vi "MAIN_HGB2_rev03.vi"() -> ()   [LabVIEW 2016]
uses:
  Producer_Case_Structure.ctl
  Consumer Control.ctl
  <vilib>/Utility/error.llb/DialogType.ctl
  <vilib>/DAQmx/write.llb/DAQmx Write (Analog 1D DBL NChan 1Samp).vi
  <vilib>/DAQmx/miscellaneous.llb/DAQmx Fill In Error Info.vi
  <vilib>/express/express analysis/Spectral/Block/exnSpectralBlock spectral measurements RMS poly.vi
  <vilib>/express/express analysis/Spectral/Block/exnSpectralBlock spectral measurements RMS array WFM.vi
  <vilib>/express/express analysis/Spectral/XNode/ExpressSpectralMeasurementsBlockNode.xnode
panel:
  in  "Dummy Variable 2":dbl=100.0
  in  "VFD On/Off":bool
  out "TDMS":i32=31
  out "Acc":i32
  in  "Numeric":i32
  out "Producer":i32=452
  out "Control":i32=10
  in  "Speed Setpoint":dbl
  in  "Operator Notes":string
  in  "Dummy Variable":dbl
  in  "Record Data":bool
  in  "Sample Rate [S/s]":dbl=10.0
  in  "file path":path=path "S:/002 - Projects/200804 AECSSB/6-Testing/TDMS Data/raw/JunkData/082621-ShutdownCheck4"
  in  "Stop":bool
  in  "Tab Control":T1(tab)=enum."Pressure & Temperature"
  out "System Temperatures":waveform(dbl)[](graph)=[{"t0"=timestamp(3712839887.203294 s since 1904-01-01), "dt"=0.1, "Y"=[25.650665015231628, 25.650665015231628, 25.650665015231628, 25.650094032394826, 25.650094032394826], "attributes"=variant("NI_ChannelName"=variant(string "T_dis_dwnstrm"), "NI_UnitDescription"=variant(string "Deg C"))}, {"t0"=timestamp(3712839887.203294 s since 1904-01-01), "dt"=0.1, "Y"=[21.37303402901582, 21.37303402901582, 21.37303402901582, 21.36692834475169, 21.36692834475169], "attributes"=variant("NI_ChannelName"=variant(string "T_liq"), "NI_UnitDescription"=variant(string "Deg C"))}, {"t0"=timestamp(3712839887.203294 s since 1904-01-01), "dt"=0.1, "Y"=[25.051178589493077, 25.051178589493077, 25.051178589493077, 25.046720547133443, 25.046720547133443], "attributes"=variant("NI_ChannelName"=variant(string "T_gas_mix"), "NI_UnitDescription"=variant(string "Deg C"))}, {"t0"=timestamp(3712839887.203294 s since 1904-01-01), "dt"=0.1, "Y"=[15.28260420449759, 15.28260420449759, 15.28260420449759, 15.302095088188059, 15.302095088188059], "attributes"=variant("NI_ChannelName"=variant(string "T_wf_cd_out"), "NI_UnitDescription"=variant(string "Deg C"))}, {"t0"=timestamp(3712839887.203294 s since 1904-01-01), "dt"=0.1, "Y"=[17.854844556084544, 17.854844556084544, 17.854844556084544, 17.936201243083087, 17.936201243083087], "attributes"=variant("NI_ChannelName"=variant(string "T_cf_in"), "NI_UnitDescription"=variant(string "Deg C"))}]
  out "System Pressures":waveform(dbl)[](graph)=[{"t0"=timestamp(3712839887.203294 s since 1904-01-01), "dt"=0.1, "Y"=[497.9062778476196, 497.9617200549117, 497.9593536192346, 497.9556349345991, 497.93366088902604], "attributes"=variant("NI_ChannelName"=variant(string "P_comp_suc"))}, {"t0"=timestamp(3712839887.203294 s since 1904-01-01), "dt"=0.1, "Y"=[500.46360622081005, 500.48118547426617, 500.5396702982644, 500.502145353387, 500.5122872303809], "attributes"=variant("NI_ChannelName"=variant(string "P_comp_dis"))}, {"t0"=timestamp(3712839887.203294 s since 1904-01-01), "dt"=0.1, "Y"=[498.7526715719359, 498.6975673736022, 498.7459103206066, 498.7313736302486, 498.67626943191505], "attributes"=variant("NI_ChannelName"=variant(string "P_comp_int"))}]
  out "Mass Flow":waveform(dbl)(graph)={"t0"=timestamp(3712839887.203294 s since 1904-01-01), "dt"=0.1, "Y"=[-2.5258889253594596e-05, -2.5376565371472426e-05, -2.545011294514607e-05, -2.5361855856737697e-05, -2.5361855856737697e-05], "attributes"=variant("NI_ChannelName"=variant(string "m_dot_wf"))}
  out "Setpoint Temperatures":waveform(dbl)[](graph)=[{"t0"=timestamp(3712839887.203294 s since 1904-01-01), "dt"=0.1, "Y"=[26.12327874474579, 26.12327874474579, 26.12327874474579, 26.12567352372733, 26.12567352372733], "attributes"=variant("NI_ChannelName"=variant(string "T_comp_suc"), "NI_UnitDescription"=variant(string "Deg C"))}, {"t0"=timestamp(3712839887.203294 s since 1904-01-01), "dt"=0.1, "Y"=[25.833285073903582, 25.833285073903582, 25.833285073903582, 25.830203756237246, 25.830203756237246], "attributes"=variant("NI_ChannelName"=variant(string "T_comp_out"), "NI_UnitDescription"=variant(string "Deg C"))}, {"t0"=timestamp(3712839887.203294 s since 1904-01-01), "dt"=0.1, "Y"=[10.549528033625506, 10.546050512616432, 10.546198937365375, 10.548826956323552, 10.550205219635103], "attributes"=variant("NI_ChannelName"=variant(string "Suc_Suph"), "NI_UnitDescription"=variant(string "Deg C"))}]
  out "Power Constituents":waveform(dbl)[](graph)=[{"t0"=timestamp(3712839887.203294 s since 1904-01-01), "dt"=0.1, "Y"=[-0.25374797068745636, -0.25404216098215215, -0.25404216098215215, -0.2541402244137174, -0.2541402244137174], "attributes"=variant("NI_ChannelName"=variant(string "Voltage"))}, {"t0"=timestamp(3712839887.203294 s since 1904-01-01), "dt"=0.1, "Y"=[-0.030598737819417465, -0.031007335450937035, -0.031203462314064012, -0.031154430598284932, -0.0311053988825023], "attributes"=variant("NI_ChannelName"=variant(string "Frequency"))}, {"t0"=timestamp(3712839886.9042945 s since 1904-01-01), "dt"=0.1, "Y"=[0.03397996537387371, 0.003032894805073738, -0.007282795384526253, -0.0021249502897262573, -0.012440640479326248], "attributes"=variant("NI_ChannelName"=variant(string "Torque"))}, {"t0"=timestamp(3712839886.9542933 s since 1904-01-01), "dt"=0.1, "Y"=[-13.228808343410492, 7.40257203578949, 1.2131579220294952, -9.102532267570496, 9.465710073709488], "attributes"=variant("NI_ChannelName"=variant(string "Tachometer"))}]
  out "Raw Acceleration":waveform(dbl)[](graph)
  out "Accel. Spectrum":cluster{"f0":dbl, "df":dbl, "magnitude":dbl[]}[](graph)
  in  "?":path=path "C:/Users/ASITest/Desktop/REFPROP"
  in  "Working Fluid":string="R134A.FLD"
  # "Stop VI"
  # "Air Squared Hot Gas Bypass Test Stand"
  # "Point to where REFPROP is..."
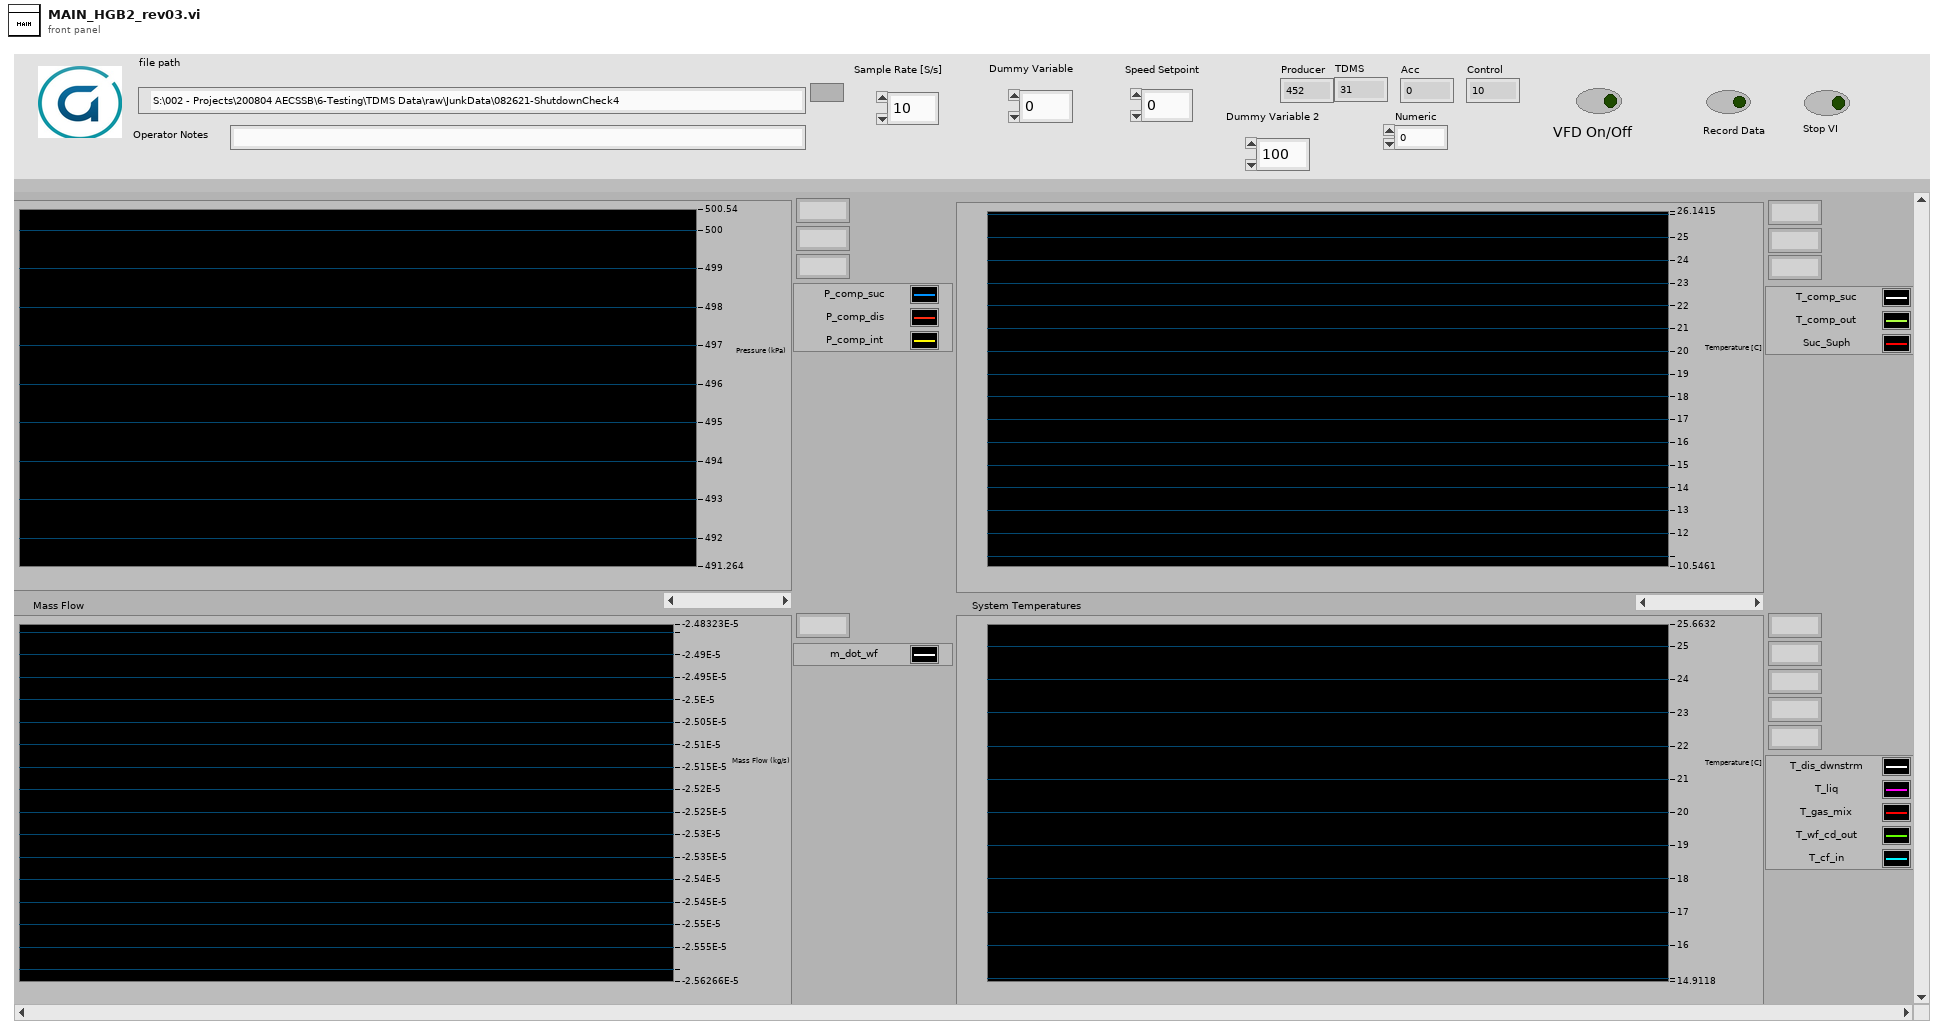
[diagram p1: front panel]
types:
  T1 = enum32{"Schematic", "Pressure & Temperature", "Power", "Acceleration", "Efficiency"}
  T2 = typedef "Consumer Control.ctl" = enum16{"System Run", "Shutdown"}
  T3 = enum16{"open", "open or create", "create or replace", "create", "open (read-only)"}
  T4 = typedef "Producer_Case_Structure.ctl" = enum16{"Initialize", "Read", "Write", "Display", "Queue", "Evaluate", "Error", "Shutdown"}
  T5 = cluster{"Data Main":waveform(dbl)[], "Accelerometer":waveform(dbl)[], "Dummy Variable":dbl, "Operator Notes":string, "Speed Setpoint":dbl, "NI 6001":waveform(dbl)[], "On/Off":dbl}
  T6 = typedef "DialogType.ctl" = u16
  T7 = cluster{"averaging mode":u16, "weighting mode":u16, "number of averages":u32}
  T8 = cluster{"dB On (F)":bool, "unwrap phase (F)":bool, "convert to degree (F)":bool}
  T9 = cluster{"All Channels":tag[], "All Labels":string[], "All Units":string[], "Slope":dbl[], "Y-Intercept":dbl[]}
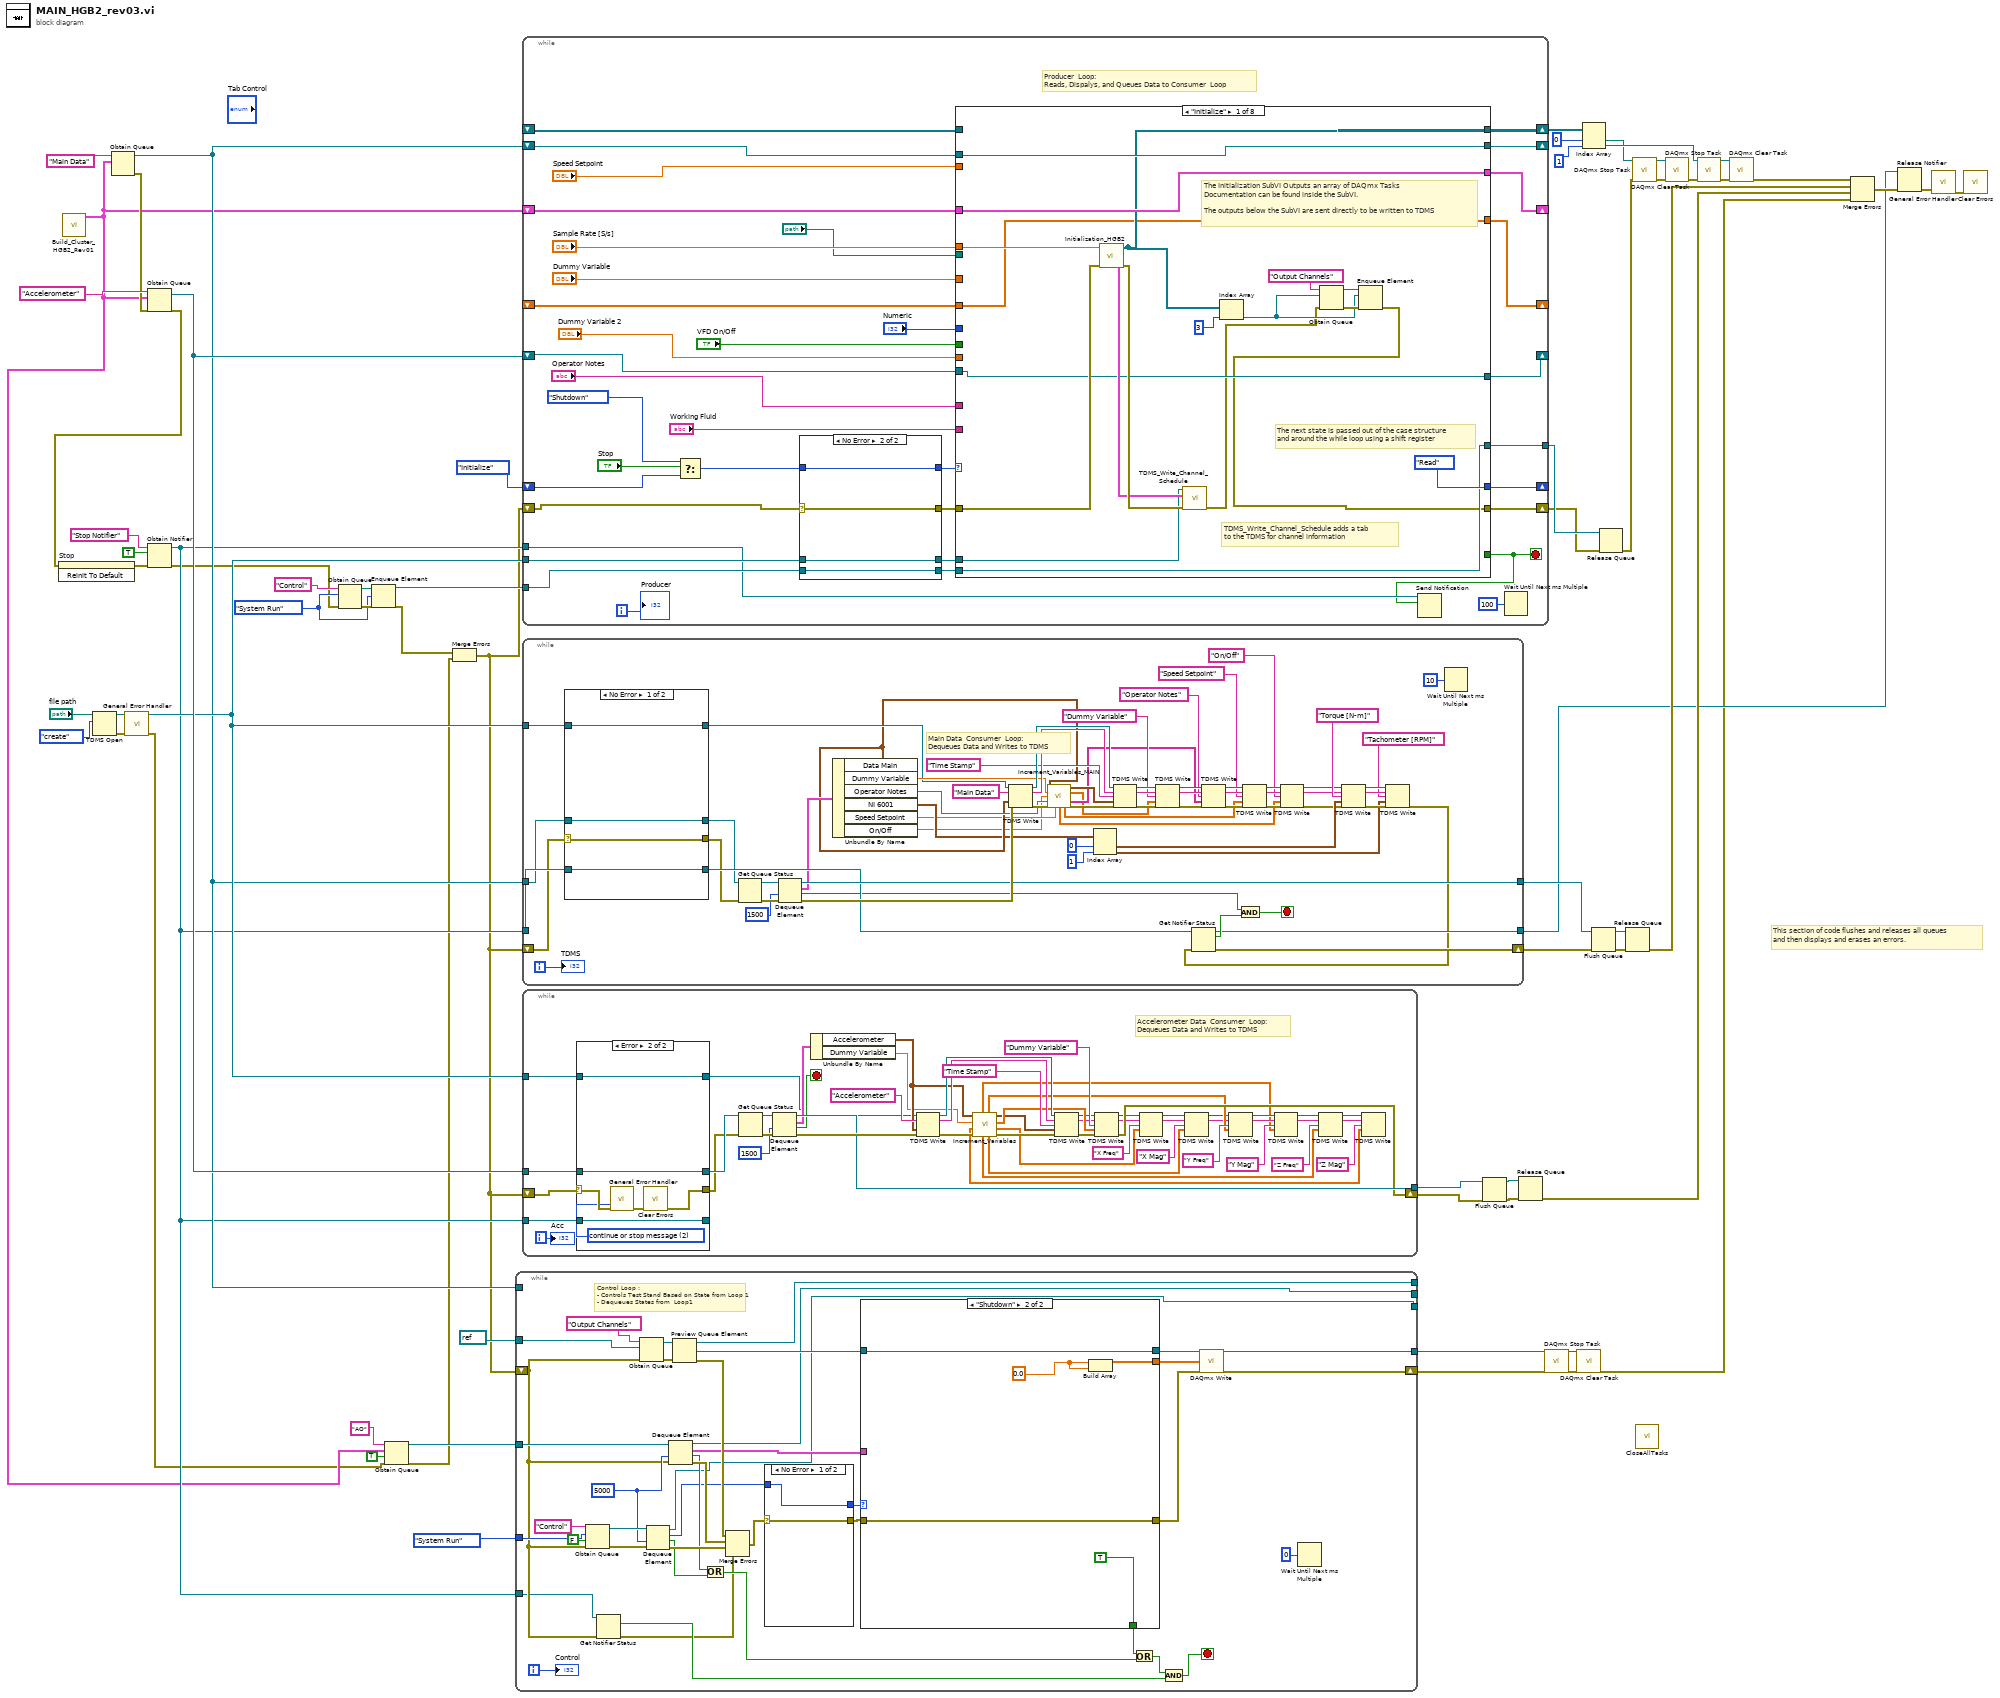
[diagram p0: block diagram]
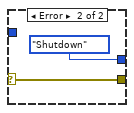
[diagram p2: hidden frame]
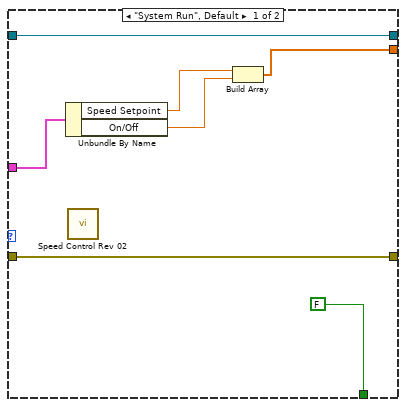
[diagram p3: hidden frame]
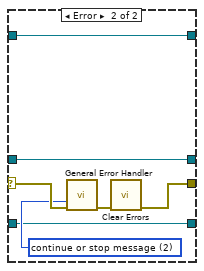
[diagram p5: hidden frame]
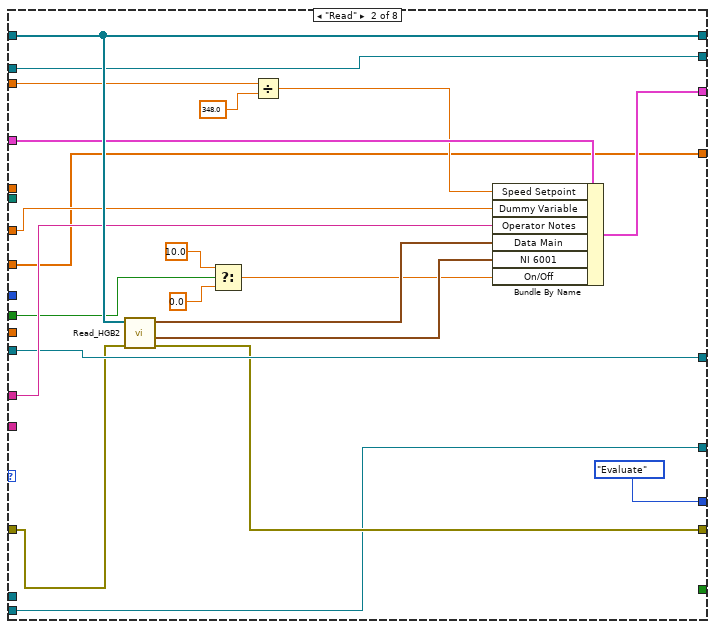
[diagram p6: hidden frame]
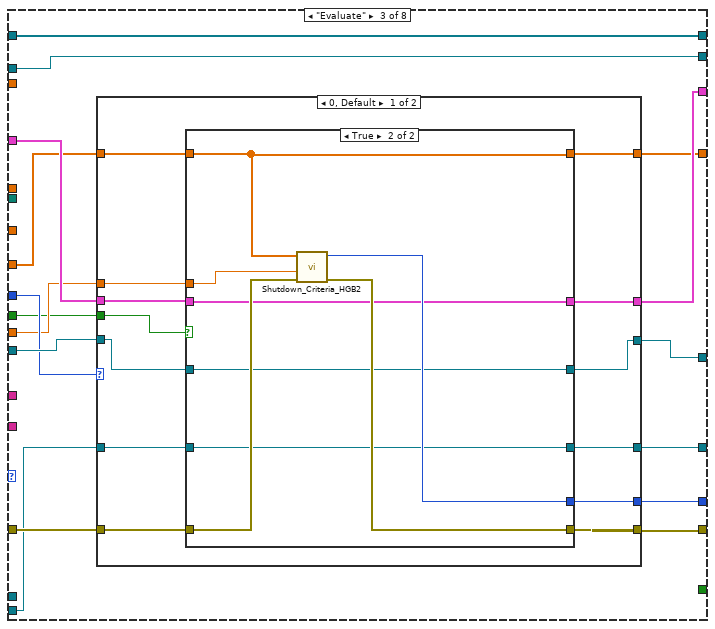
[diagram p7: hidden frame]
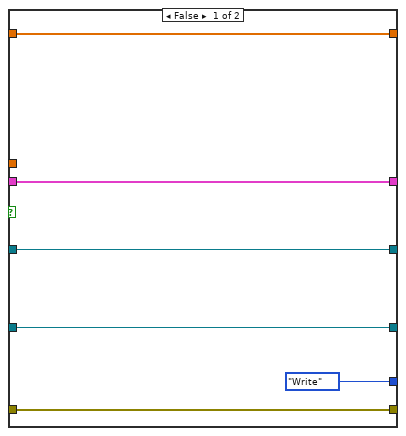
[diagram p8: hidden frame]
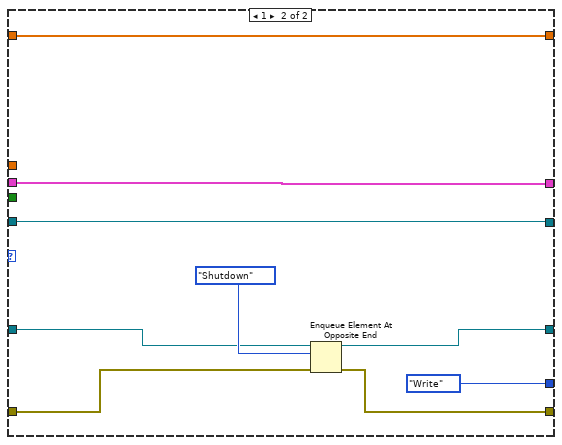
[diagram p9: hidden frame]
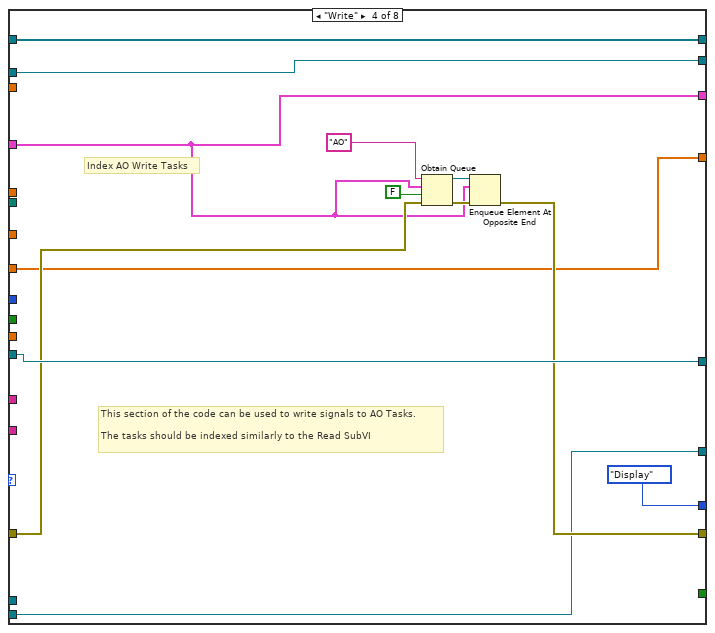
[diagram p10: hidden frame]
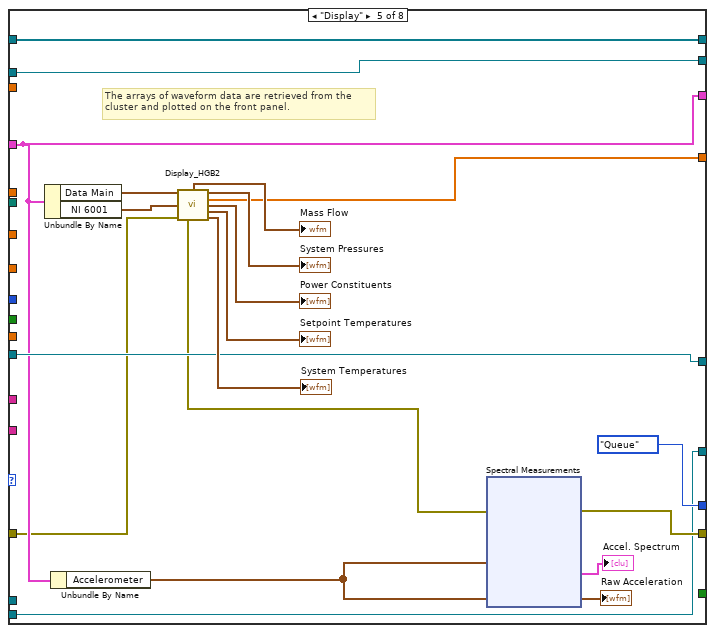
[diagram p11: hidden frame]
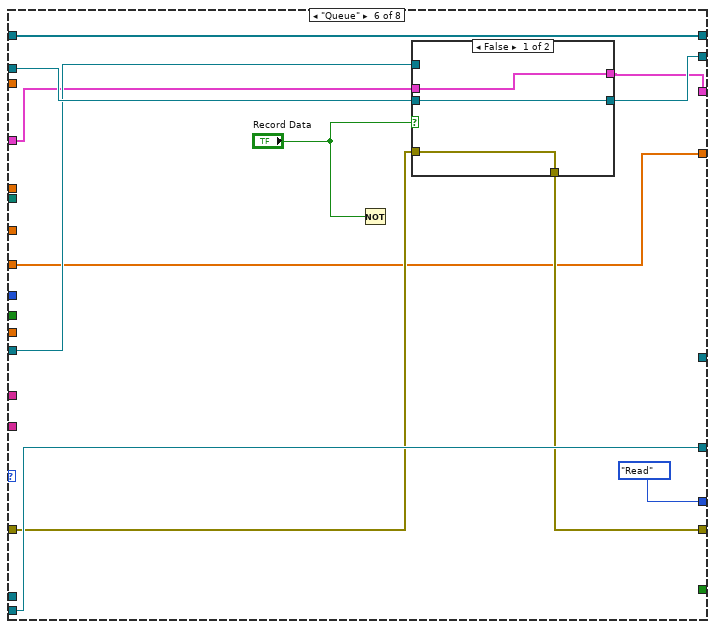
[diagram p12: hidden frame]
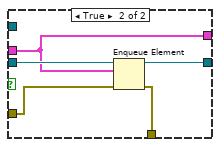
[diagram p13: hidden frame]
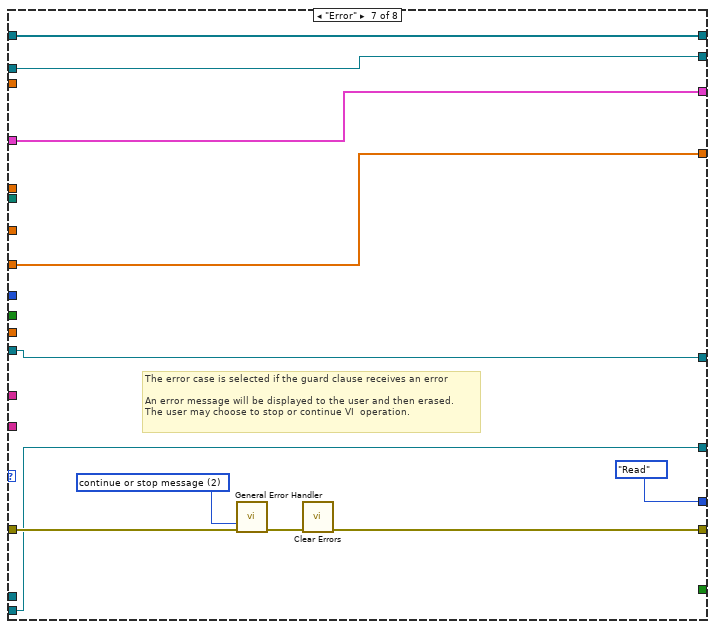
[diagram p14: hidden frame]
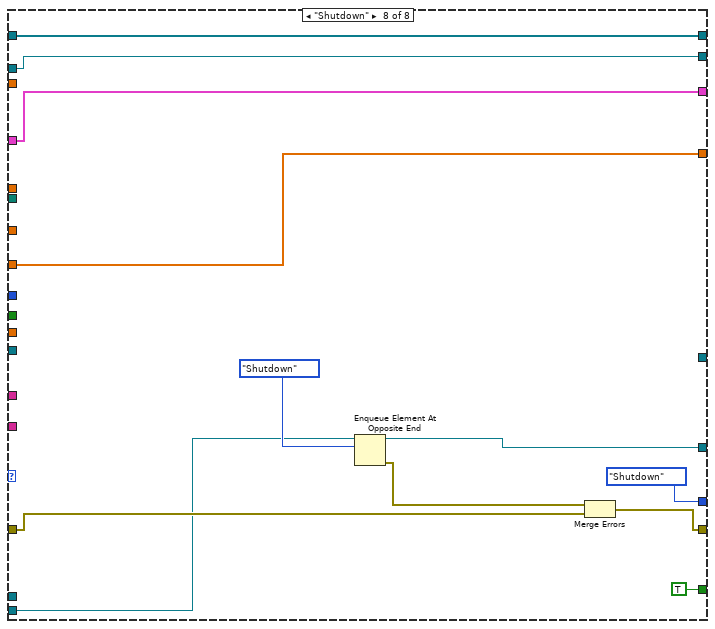
[diagram p15: hidden frame]
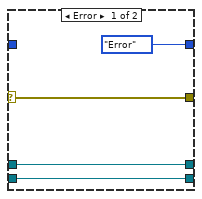
[diagram p16: hidden frame]
diagram:
  w21 = Consumer_Control."System Run"
  # "This section of code flushes and releases all queues \nand then displays and erases an errors."
  n1 = call "Build_Cluster_HGB2_Rev01.vi"() -> ("output cluster"=w13:T5)  [unwired: 11 in]
  n2 = TDMS Open(10:T3."create" ("operation (0:open)"), 11:"file path") -> (0:w54:errorcluster, 3:w37:refnum<k34>)  [unwired: 5 in]
  n3 = Obtain Queue(name (unnamed)="Main Data", element data type=w13) -> (queue out=w34:refnum<queue>, error out=w43:errorcluster)  [unwired: 3 in, 1 out]
  n4 = call <vilib>:"General Error Handler.vi"("error in (no error)"=w54) -> ("error out"=w12:errorcluster)  [unwired: 10 in, 4 out]
  n5 = Obtain Queue(name (unnamed)="Accelerometer", element data type=w13, error in (no error)=w43) -> (queue out=w42:refnum<queue>, error out=w11:errorcluster)  [unwired: 2 in, 1 out]
  n6 = invoke on="Stop" class="Bool (strict)" method="Reinit To Default"(error in=w11) -> (error out=w59:errorcluster)  [unwired: 2 in, 2 out]
  n7 = Obtain Notifier(name (unnamed)="Stop Notifier", notification data type=TRUE, error in (no error)=w59) -> (notifier out=w30:refnum<notifier>, error out=w10:errorcluster)  [unwired: 1 in, 1 out]
  n8 = Obtain Queue(name (unnamed)="Control", element data type=w21, error in (no error)=w10) -> (queue out=w23:refnum<queue>, error out=w22:errorcluster)  [unwired: 2 in, 1 out]
  n9 = Enqueue Element(queue=w23, element=w21, error in (no error)=w22) -> (queue out=w20:refnum<queue>, error out=w8:errorcluster)  [unwired: 1 in, 1 out]
  n10 = Obtain Queue(name (unnamed)="AO", element data type=w13, create if not found? (T)=TRUE, error in (no error)=w12) -> (queue out=w14:refnum<queue>, error out=w7:errorcluster)  [unwired: 1 in, 1 out]
  n11 = Merge Errors(w8, w7) -> (w9:errorcluster)
  n12 = while {
    tunnel: [w102] -> w4
    shift-right: [w89] -> w3
    shift-left: w9 -> [w70]
    tunnel: refnum<k21> refnum ("task in") -> [w97]
    tunnel: w34 -> [_]
    tunnel: Consumer_Control."System Run" -> [w87]
    tunnel: w30 -> [w69]
    tunnel: [w74] -> _
    tunnel: [w73] -> _
    tunnel: [w72] -> _
    tunnel: w14 -> [w71]
    i -> [w79]
    stop <- w68 stop-if-true
    w92 = 5000 ("timeout in ms (-1)")
    # "Control Loop :\n- Controls Test Stand Based on State from Loop 1\n- Dequeues States from  Loop1"
    n13 = Obtain Queue(name (unnamed)="Control", element data type=w87, create if not found? (T)=FALSE, error in (no error)=w70) -> (queue out=w101:refnum<queue>, error out=w93:errorcluster)  [unwired: 1 in, 1 out]
    n14 = Get Notifier Status(notifier=w69, error in (no error)=w70) -> (current notification=w66:bool, error out=w65:errorcluster)  [unwired: 3 out]
    n15 = Obtain Queue(name (unnamed)="Output Channels", element data type=w97, error in (no error)=w70) -> (queue out=w98:refnum<queue>, error out=w96:errorcluster)  [unwired: 2 in, 1 out]
    n16 = Dequeue Element(queue=w101, timeout in ms (-1)=w92, error in (no error)=w93) -> (queue out=w72:refnum<queue>, element=w86:T2, timed out?=w90:bool, error out=w94:errorcluster)
    n17 = Dequeue Element(queue=w71, timeout in ms (-1)=w92, error in (no error)=w70) -> (queue out=w73:refnum<queue>, element=w80:T5, timed out?=w91:bool, error out=w95:errorcluster)
    n18 = Preview Queue Element(queue=w98, error in (no error)=w96) -> (queue out=w74:refnum<queue>, element=w99:refnum<k21>, error out=w88:errorcluster)  [unwired: 1 in, 1 out]
    n19 = Or(x=w91, y=w90) -> (x .or. y?=w77:bool)
    n20 = Merge Errors(w88, w95, w94, w65) -> (w85:errorcluster)
    n21 = case shown="No Error" w85 {
      selector: w85 -> [w106 w108]
      tunnel: [w106 w108] -> w84
      tunnel: w86 -> [w105 _]
      tunnel: [w105 Consumer_Control."Shutdown"] -> w83
      frame No Error {
      }
      frame Error {
      }
    }
    n22 = case shown="\"Shutdown\"" w83 {
      tunnel: w99 -> [w115 w119]
      tunnel: [w110 w120] -> w104
      tunnel: [w115 w119] -> w103
      tunnel: w80 -> [w112 _]
      tunnel: w84 -> [w113 w117]
      tunnel: [FALSE TRUE] -> w78
      tunnel: [w113 w117] -> w82
      frame "System Run", Default {
        n23 = Unbundle By Name(w112) -> ("Speed Setpoint"=w111:dbl, "On/Off"=w109:dbl)
        n24 = call "Speed Control Rev 02.vi"() -> ()  [unwired: 11 in, 1 out]
        n25 = Build Array(w111, w109) -> (w110:dbl[])
      }
      frame "Shutdown" {
        w116 = 0.0 ("Speed Setpoint 2")
        n26 = Build Array(w116, w116) -> (w120:dbl[])
      }
    }
    n27 = Or(x=w78, y=w77) -> (x .or. y?=w67:bool)
    n28 = And(x=w67, y=w66) -> (x .and. y?=w68:bool)
    n29 = call-poly <vilib>:"DAQmx Write.vi"("task/channels in"=w103, "data"=w104, "error in"=w82) -> ("task out"=w102:refnum<k21>, "error out"=w89:errorcluster)  [unwired: 10 in, 1 out]
    n30 = Wait Until Next ms Multiple(millisecond multiple=u32 0) -> ()  [unwired: 1 out]
    "Control" <- w79
  }
  n31 = while {
    tunnel: w37 -> [w175]
    tunnel: [w185] -> w51
    tunnel: w34 -> [w176]
    tunnel: w30 -> [w178]
    shift-right: [w183] -> w26
    shift-left: w9 -> [w174]
    tunnel: [w153] -> w25
    i -> [w138]
    stop <- w180 stop-if-true
    # "Main Data  Consumer  Loop: \nDequeues Data and Writes to TDMS"
    n32 = case shown="No Error" w174 {
      selector: w174 -> [w191 w197]
      tunnel: [w191 w196] -> w156
      tunnel: w178 -> [w190 w192]
      tunnel: [w190 w192] -> w179
      tunnel: [w189 w194] -> w177
      tunnel: w176 -> [w189 w194]
      tunnel: [w188 w193] -> w154
      tunnel: w175 -> [w188 w193]
      frame No Error {
      }
      frame Error {
        w195 = T6 2 items=["no dialog", "OK message", "continue or stop message", "OK message + warnings", "continue/stop + warnings"] ("type of dialog (OK msg:1)")
        n33 = call <vilib>:"General Error Handler.vi"("type of dialog (OK msg:1)"=w195, "error in (no error)"=w197) -> ("error out"=w198:errorcluster)  [unwired: 9 in, 4 out]
        n34 = call <vilib>:"Clear Errors.vi"("error in (no error)"=w198) -> ("error out"=w196:errorcluster)  [unwired: 5 in, 1 out]
      }
    }
    n35 = Get Queue Status(queue=w177, error in (no error)=w156) -> (queue out=w182:refnum<queue>, error out=w186:errorcluster)  [unwired: 1 in, 6 out]
    n36 = Dequeue Element(queue=w182, timeout in ms (-1)=1500, error in (no error)=w186) -> (queue out=w185:refnum<queue>, element=w155:T5, timed out?=w173:bool, error out=w187:errorcluster)
    n37 = Unbundle By Name(w155) -> ("Data Main"=w145:waveform(dbl)[], "Dummy Variable"=w163:dbl, "Operator Notes"=w151:string, "NI 6001"=w140:waveform(dbl)[], "Speed Setpoint"=w139:dbl, "On/Off"=w123:dbl)
    n38 = TDMS Write(0:w154, 5:"Main Data" ("group name in (Untitled)"), 9:w145, 11:w187) -> (4:w170:refnum<k34>, 6:w168:string, 15:w171:errorcluster)  [unwired: 2 in, 1 out]
    n39 = call "Increment_Variables_MAIN.vi"("Data Main"=w145, "Dummy Variable"=w163, "On/Off"=w123, "Operator Notes"=w151, "error in 2"=w171, "Speed Setpoint"=w139) -> ("Time Stamp"=w164:timestamp[], "Dummy Variable Array"=w141:dbl[], "Operator Notes Array"=w152:string[], "On/Off Array"=w122:dbl[], "Speed Setpoint Array"=w147:dbl[], "error IO"=w172:errorcluster)  [unwired: 4 in]
    n40 = Index Array(array=w140, index #1=0 ("index"), index #2=1 ("index")) -> (element #1=w142:waveform(dbl), element #2=w130:waveform(dbl))
    n41 = TDMS Write(0:w170, 5:w168, 7:"Time Stamp" ("group name in (Untitled)"), 9:w164, 11:w172) -> (4:w167:refnum<k34>, 6:w165:string, 15:w166:errorcluster)  [unwired: 1 in, 1 out]
    n42 = TDMS Write(0:w167, 5:w165, 7:"Dummy Variable" ("group name in (Untitled)"), 9:w141, 11:w166) -> (4:w161:refnum<k34>, 6:w160:string, 15:w162:errorcluster)  [unwired: 1 in, 1 out]
    n43 = TDMS Write(0:w161, 5:w160, 7:"Operator Notes" ("group name in (Untitled)"), 9:w152, 11:w162) -> (4:w148:refnum<k34>, 6:w149:string, 15:w150:errorcluster)  [unwired: 1 in, 1 out]
    n44 = TDMS Write(0:w148, 5:w149, 7:"Speed Setpoint" ("group name in (Untitled)"), 9:w147, 11:w150) -> (4:w129:refnum<k34>, 6:w128:string, 15:w127:errorcluster)  [unwired: 1 in, 1 out]
    n45 = TDMS Write(0:w129, 5:w128, 7:"On/Off" ("channel name(s) in (Untitled)"), 9:w122, 11:w127) -> (4:w125:refnum<k34>, 6:w124:string, 15:w126:errorcluster)  [unwired: 1 in, 1 out]
    n46 = TDMS Write(0:w125, 5:w124, 7:"Torque [N-m]" ("channel name(s) in (Untitled)"), 9:w142, 11:w126) -> (4:w132:refnum<k34>, 6:w133:string, 15:w135:errorcluster)  [unwired: 1 in, 1 out]
    n47 = TDMS Write(0:w132, 5:w133, 7:"Tachometer [RPM]" ("channel name(s) in (Untitled)"), 9:w130, 11:w135) -> (15:w134:errorcluster)  [unwired: 1 in, 3 out]
    n48 = Get Notifier Status(notifier=w179, error in (no error)=w134) -> (notifier out=w153:refnum<notifier>, current notification=w184:bool, error out=w183:errorcluster)  [unwired: 2 out]
    n49 = And(x=w173, y=w184) -> (x .and. y?=w180:bool)
    n50 = Wait Until Next ms Multiple(millisecond multiple=u32 10) -> ()  [unwired: 1 out]
    "TDMS" <- w138
  }
  n51 = while {
    shift-right: [w230] -> _
    shift-left: Producer_Case_Structure."Initialize" ("Enum") -> [w209]
    shift-right: [w232] -> w56
    shift-left: _ -> [w231]
    tunnel: w30 -> [w206]
    shift-right: [w229] -> _
    shift-left: w13 -> [w228]
    shift-right: [w227] -> _
    shift-left: w34 -> [w226]
    shift-right: [w233] -> w18
    shift-left: w9 -> [w205]
    tunnel: w37 -> [w221]
    shift-right: [w219] -> _
    shift-left: w42 -> [w220]
    tunnel: w20 -> [w214]
    tunnel: [w212] -> w19
    shift-right: [w202] -> _
    shift-left: _ -> [w201]
    i -> [w215]
    stop <- w199 stop-if-true
    # "Producer  Loop: \nReads, Dispalys, and Queues Data to Consumer  Loop"
    n52 = Select(t=Producer_Case_Structure."Shutdown" ("Enum"), s="Stop", f=w209) -> (s? t:f=w208:T4)
    n53 = case shown="No Error" w205 {
      selector: w205 -> [w415 w420]
      tunnel: [w415 w420] -> w234
      tunnel: w208 -> [_ w419]
      tunnel: [Producer_Case_Structure."Error" ("Enum") w419] -> w235
      tunnel: [w414 w418] -> w222
      tunnel: w221 -> [w414 w418]
      tunnel: w214 -> [w413 w417]
      tunnel: [w413 w417] -> w213
      frame Error {
      }
      frame No Error {
      }
    }
    n54 = case shown="\"Initialize\"" w235 {
      tunnel: w234 -> [w254 w263 w289 w334 w344 w372 w397 w410]
      tunnel: [w237 w266 w288 w336 w352 w371 w394 w409] -> w233
      tunnel: [w242 w274 w284 w340 w358 w380 w398 w406] -> w232
      tunnel: w231 -> [_ w274 w284 w340 w358 w380 w398 w406]
      tunnel: [Producer_Case_Structure."Read" ("Enum") Producer_Case_Structure."Evaluate" ("Enum") w280 Producer_Case_Structure."Display" ("Enum") Producer_Case_Structure."Queue" ("Enum") Producer_Case_Structure."Read" ("Enum") Producer_Case_Structure."Read" ("Enum") Producer_Case_Structure."Shutdown" ("Enum")] -> w230
      tunnel: [_ _ _ _ _ _ _ TRUE ("Stop")] -> w199
      tunnel: [w250 w272 w290 w329 w351 w377 w396 w404] -> w229
      tunnel: w228 -> [w250 w268 w291 w329 w351 w375 w396 w404]
      tunnel: [w252 w273 w285 w338 w356 w378 w393 w405] -> w227
      tunnel: w226 -> [w252 w273 w285 w338 w356 w379 w393 w405]
      tunnel: "Sample Rate [S/s]" -> [w251 _ _ _ _ _ _ _]
      tunnel: "Dummy Variable" -> [_ w269 _ _ _ _ _ _]
      tunnel: "Operator Notes" -> [_ w271 _ _ _ _ _ _]
      tunnel: w222 -> [w247 _ _ _ _ _ _ _]
      tunnel: w220 -> [w246 w270 w283 w337 w354 w376 w392 _]
      tunnel: [w246 w270 w282 w337 w354 _ w392 _] -> w219
      tunnel: "?" -> [_ _ _ _ _ _ _ _]
      tunnel: "Working Fluid" -> [_ _ _ _ _ _ _ _]
      tunnel: "Speed Setpoint" -> [_ w257 _ _ _ _ _ _]
      tunnel: w213 -> [w239 w264 w287 w335 w343 w373 w391 w408]
      tunnel: [w239 w264 w286 w335 w343 w373 w391 w407] -> w212
      tunnel: "Numeric" -> [_ _ w281 _ _ _ _ _]
      tunnel: "VFD On/Off" -> [_ w260 w276 _ _ _ _ _]
      tunnel: [w236 w255 w278 w328 w342 w370 w390 w401] -> w202
      tunnel: w201 -> [w236 w255 w279 w328 _ w370 w390 w401]
      tunnel: "Dummy Variable 2" -> [_ _ w277 _ _ _ _ _]
      frame "Initialize" {
        # "TDMS_Write_Channel_Schedule adds a tab \nto the TDMS for channel information"
        # "The next state is passed out of the case structure \nand around the while loop using a shift register"
        # "The Initialization SubVI Outputs an array of DAQmx Tasks\nDocumentation can be found inside the SubVI.\n\nThe outputs below the SubVI are sent directly to be written to TDMS"
        n55 = call "Initialization_HGB2.vi"("error in"=w254, "Sample Rate"=w251) -> ("error out"=w249:errorcluster, "Task Array"=w242:refnum<k21>[], "output cluster"=w248:T9)  [unwired: 7 in]
        n56 = call "TDMS_Write_Channel_Schedule.vi"("error in (no error)"=w249, "output cluster"=w248, "Refnum in"=w247) -> ("error out"=w238:errorcluster)  [unwired: 8 in]
        n57 = Index Array(array=w242, index=3) -> (element=w240:refnum<k21>)
        n58 = Obtain Queue(name (unnamed)="Output Channels", element data type=w240, error in (no error)=w238) -> (queue out=w244:refnum<queue>, error out=w243:errorcluster)  [unwired: 2 in, 1 out]
        n59 = Enqueue Element(queue=w244, element=w240, error in (no error)=w243) -> (error out=w237:errorcluster)  [unwired: 1 in, 2 out]
      }
      frame "Read" {
        n60 = call "Read_HGB2.vi"("error in (no error)"=w263, "Task Array"=w274) -> ("error out"=w266:errorcluster, "NI 6001"=w265:waveform(dbl)[], "Data Main"=w267:waveform(dbl)[])  [unwired: 7 in]
        n61 = Select(t=10.0, s=w260, f=0.0) -> (s? t:f=w259:dbl)
        n62 = Divide(x=w257, y=348.0) -> (x/y=w256:dbl)
        n63 = Bundle By Name(cluster=w268, "Speed Setpoint"=w256, "Dummy Variable"=w269, "Operator Notes"=w271, "Data Main"=w267, "NI 6001"=w265, "On/Off"=w259) -> (w272:T5)
      }
      frame "Evaluate" {
        n64 = case shown="0, Default" w281 {
          tunnel: w291 -> [w300 w327]
          tunnel: [w299 w327] -> w290
          tunnel: w289 -> [w304 w323]
          tunnel: [w302 w322] -> w288
          tunnel: w287 -> [w293 w325]
          tunnel: [w292 w324] -> w286
          tunnel: [w298 w321] -> w282
          tunnel: w283 -> [w297 w321]
          tunnel: [w301 Producer_Case_Structure."Write" ("Enum")] -> w280
          tunnel: w279 -> [w294 w319]
          tunnel: [w295 w319] -> w278
          tunnel: w277 -> [w303 _]
          tunnel: w276 -> [w296 _]
          frame 0, Default {
            n65 = case shown="True" w296 {
              tunnel: w294 -> [w310 w312]
              tunnel: w304 -> [w307 w318]
              tunnel: w303 -> [_ w317]
              tunnel: [w307 w316] -> w302
              tunnel: [Producer_Case_Structure."Write" ("Enum") w315] -> w301
              tunnel: w300 -> [w309 w314]
              tunnel: [w309 w314] -> w299
              tunnel: [w308 w313] -> w298
              tunnel: w297 -> [w308 w313]
              tunnel: [w310 w312] -> w295
              tunnel: w293 -> [w306 w311]
              tunnel: [w306 w311] -> w292
              frame False {
              }
              frame True {
                n66 = call "Shutdown_Criteria_HGB2.vi"("error in (no error)"=w318, "Dummy Variable 2"=w317, "Data Array"=w312) -> ("error out"=w316:errorcluster, "Enum"=w315:T4)  [unwired: 7 in]
              }
            }
          }
          frame 1 {
            n67 = Enqueue Element At Opposite End(queue=w325, element=Consumer_Control."Shutdown", error in (no error)=w323) -> (queue out=w324:refnum<queue>, error out=w322:errorcluster)  [unwired: 1 in, 1 out]
          }
        }
      }
      frame "Write" {
        # "This section of the code can be used to write signals to AO Tasks.\n\nThe tasks should be indexed similarly to the Read SubVI"
        # "Index AO Write Tasks"
        n68 = Obtain Queue(name (unnamed)="AO", element data type=w329, create if not found? (T)=FALSE, error in (no error)=w334) -> (queue out=w332:refnum<queue>, error out=w333:errorcluster)  [unwired: 1 in, 1 out]
        n69 = Enqueue Element At Opposite End(queue=w332, element=w329, error in (no error)=w333) -> (error out=w336:errorcluster)  [unwired: 1 in, 2 out]
      }
      frame "Display" {
        # "The arrays of waveform data are retrieved from the \ncluster and plotted on the front panel."
        n70 = Unbundle By Name(w351) -> ("Data Main"=w349:waveform(dbl)[], "NI 6001"=w345:waveform(dbl)[])
        n71 = Unbundle By Name(w351) -> ("Accelerometer"=w350:waveform(dbl)[])
        "Raw Acceleration" <- w350
        n72 = call "Display_HGB2.vi"("data"=w349, "NI 6001"=w345, "error in (no error)"=w344) -> ("Mass Flow"=→"Mass Flow":waveform(dbl), "System Pressures"=→"System Pressures":waveform(dbl)[], "Data Array"=w342:dbl[], "Power Constituents"=→"Power Constituents":waveform(dbl)[], "Setpoint Temperatures"=→"Setpoint Temperatures":waveform(dbl)[], "error out"=w353:errorcluster, "System Temperatures"=→"System Temperatures":waveform(dbl)[])  [unwired: 6 in]
        n73 = xnode "Spectral Measurements"("Signals"=w350, "error in (no error)"=w353) -> ("FFT - (RMS)"=→"Accel. Spectrum":cluster{"f0":dbl, "df":dbl, "magnitude":dbl[]}[], "error out"=w352:errorcluster)  [unwired: 1 out]
      }
      frame "Queue" {
        n74 = Not(x="Record Data") -> ()  [unwired: 1 out]
        n75 = case shown="False" "Record Data" {
          tunnel: w375 -> [w383 w387]
          tunnel: w379 -> [w384 w388]
          tunnel: [w384 w389] -> w378
          tunnel: [w383 w387] -> w377
          tunnel: w376 -> [_ _]
          tunnel: w372 -> [w382 w386]
          tunnel: [w382 w385] -> w371
          frame False {
          }
          frame True {
            n76 = Enqueue Element(queue=w388, element=w387, error in (no error)=w386) -> (queue out=w389:refnum<queue>, error out=w385:errorcluster)  [unwired: 1 in, 1 out]
          }
        }
      }
      frame "Error" {
        w399 = T6 2 items=["no dialog", "OK message", "continue or stop message", "OK message + warnings", "continue/stop + warnings"] ("type of dialog (OK msg:1)")
        # "The error case is selected if the guard clause receives an error\n\nAn error message will be displayed to the user and then erased. \nThe user may choose to stop or continue VI  operation."
        n77 = call <vilib>:"General Error Handler.vi"("type of dialog (OK msg:1)"=w399, "error in (no error)"=w397) -> ("error out"=w395:errorcluster)  [unwired: 9 in, 4 out]
        n78 = call <vilib>:"Clear Errors.vi"("error in (no error)"=w395) -> ("error out"=w394:errorcluster)  [unwired: 5 in, 1 out]
      }
      frame "Shutdown" {
        n79 = Enqueue Element At Opposite End(queue=w408, element=Consumer_Control."Shutdown") -> (queue out=w407:refnum<queue>, error out=w411:errorcluster)  [unwired: 2 in, 1 out]
        n80 = Merge Errors(w411, w410) -> (w409:errorcluster)
      }
    }
    n81 = Send Notification(notification=w199, notifier=w206) -> ()  [unwired: 1 in, 2 out]
    n82 = Wait Until Next ms Multiple(millisecond multiple=u32 100) -> ()  [unwired: 1 out]
    "Producer" <- w215
  }
  n83 = while {
    tunnel: w37 -> [w466]
    tunnel: [w472] -> w39
    tunnel: w42 -> [w467]
    tunnel: w30 -> [w469]
    shift-right: [w447] -> w36
    shift-left: w9 -> [w465]
    i -> [w421]
    stop <- w446 stop-if-true
    # "Accelerometer Data  Consumer  Loop: \nDequeues Data and Writes to TDMS"
    n84 = case shown="Error" w465 {
      selector: w465 -> [w478 w484]
      tunnel: [w478 w483] -> w457
      tunnel: w469 -> [w477 w479]
      tunnel: [w477 w479] -> _
      tunnel: [w476 w481] -> w468
      tunnel: w467 -> [w476 w481]
      tunnel: [w475 w480] -> w455
      tunnel: w466 -> [w475 w480]
      frame No Error {
      }
      frame Error {
        w482 = T6 2 items=["no dialog", "OK message", "continue or stop message", "OK message + warnings", "continue/stop + warnings"] ("type of dialog (OK msg:1)")
        n85 = call <vilib>:"General Error Handler.vi"("type of dialog (OK msg:1)"=w482, "error in (no error)"=w484) -> ("error out"=w485:errorcluster)  [unwired: 9 in, 4 out]
        n86 = call <vilib>:"Clear Errors.vi"("error in (no error)"=w485) -> ("error out"=w483:errorcluster)  [unwired: 5 in, 1 out]
      }
    }
    n87 = Get Queue Status(queue=w468, error in (no error)=w457) -> (queue out=w471:refnum<queue>, error out=w473:errorcluster)  [unwired: 1 in, 6 out]
    n88 = Dequeue Element(queue=w471, timeout in ms (-1)=1500, error in (no error)=w473) -> (queue out=w472:refnum<queue>, element=w456:T5, timed out?=w446:bool, error out=w474:errorcluster)
    n89 = Unbundle By Name(w456) -> ("Accelerometer"=w459:waveform(dbl)[], "Dummy Variable"=w454:dbl)
    n90 = TDMS Write(0:w455, 5:"Accelerometer" ("group name in (Untitled)"), 9:w459, 11:w474) -> (4:w462:refnum<k34>, 6:w460:string, 15:w463:errorcluster)  [unwired: 2 in, 1 out]
    n91 = call "Increment_Variables.vi"("error in 2"=w463, "Dummy Variable"=w454, "Accelerometer"=w459) -> ("error IO"=w464:errorcluster, "X Accel Freq Array"=w443:dbl[], "Dummy Variable Array"=w452:dbl[], "Time Stamp"=w448:timestamp[], "X Accel Mag Array"=w441:dbl[], "Y Accel Freq Array"=w424:dbl[], "Z Accel Freq Array"=w426:dbl[], "Y Accel Mag Array"=w425:dbl[], "Z Accel Mag Array"=w427:dbl[])
    n92 = TDMS Write(0:w462, 5:w460, 7:"Time Stamp" ("group name in (Untitled)"), 9:w448, 11:w464) -> (4:w449:refnum<k34>, 6:w450:string, 15:w453:errorcluster)  [unwired: 1 in, 1 out]
    n93 = TDMS Write(0:w449, 5:w450, 7:"Dummy Variable" ("group name in (Untitled)"), 9:w452, 11:w453) -> (4:w444:refnum<k34>, 6:w445:string, 15:w447:errorcluster)  [unwired: 1 in, 1 out]
    n94 = TDMS Write(0:w444, 5:w445, 7:"X Freq" ("group name in (Untitled)"), 9:w443) -> (4:w438:refnum<k34>, 6:w439:string)  [unwired: 2 in, 2 out]
    n95 = TDMS Write(0:w438, 5:w439, 7:"X Mag" ("group name in (Untitled)"), 9:w441) -> (4:w423:refnum<k34>, 6:w422:string)  [unwired: 2 in, 2 out]
    n96 = TDMS Write(0:w423, 5:w422, 7:"Y Freq" ("group name in (Untitled)"), 9:w424) -> (4:w435:refnum<k34>, 6:w434:string)  [unwired: 2 in, 2 out]
    n97 = TDMS Write(0:w435, 5:w434, 7:"Y Mag" ("group name in (Untitled)"), 9:w425) -> (4:w436:refnum<k34>, 6:w437:string)  [unwired: 2 in, 2 out]
    n98 = TDMS Write(0:w436, 5:w437, 7:"Z Freq" ("group name in (Untitled)"), 9:w426) -> (4:w433:refnum<k34>, 6:w432:string)  [unwired: 2 in, 2 out]
    n99 = TDMS Write(0:w433, 5:w432, 7:"Z Mag" ("group name in (Untitled)"), 9:w427) -> ()  [unwired: 2 in, 4 out]
    "Acc" <- w421
  }
  n100 = Flush Queue(queue=w39, error in (no error)=w36) -> (queue out=w41:refnum<queue>, error out=w40:errorcluster)  [unwired: 1 out]
  n101 = Release Queue(queue=w41, error in (no error)=w40) -> (error out=w31:errorcluster)  [unwired: 1 in, 2 out]
  n102 = call <vilib>:"DAQmx Stop Task.vi"("task/channels in"=w4, "error in"=w3) -> ("task out"=w5:refnum<k21>, "error out"=w1:errorcluster)  [unwired: 12 in]
  n103 = call <vilib>:"DAQmx Clear Task.vi"("task in"=w5, "error in"=w1) -> ("error out"=w2:errorcluster)  [unwired: 13 in]
  n104 = Index Array(array=w56, index #1=0 ("index"), index #2=1 ("index")) -> (element #1=w35:refnum<k21>, element #2=w47:refnum<k21>)
  n105 = Flush Queue(queue=w51, error in (no error)=w26) -> (queue out=w52:refnum<queue>, error out=w50:errorcluster)  [unwired: 1 out]
  n106 = Release Queue(queue=w19, error in (no error)=w18) -> (error out=w17:errorcluster)  [unwired: 1 in, 2 out]
  n107 = Release Queue(queue=w52, error in (no error)=w50) -> (error out=w32:errorcluster)  [unwired: 1 in, 2 out]
  n108 = call <vilib>:"DAQmx Stop Task.vi"("task/channels in"=w35, "error in"=w17) -> ("task out"=w57:refnum<k21>, "error out"=w58:errorcluster)  [unwired: 12 in]
  n109 = call "CloseAllTasks.vi"() -> ()  [unwired: 10 in, 1 out]
  n110 = call <vilib>:"DAQmx Clear Task.vi"("task in"=w57, "error in"=w58) -> ("error out"=w48:errorcluster)  [unwired: 13 in]
  n111 = call <vilib>:"DAQmx Stop Task.vi"("task/channels in"=w47, "error in"=w48) -> ("task out"=w45:refnum<k21>, "error out"=w49:errorcluster)  [unwired: 12 in]
  n112 = call <vilib>:"DAQmx Clear Task.vi"("task in"=w45, "error in"=w49) -> ("error out"=w6:errorcluster)  [unwired: 13 in]
  n113 = Merge Errors(w6, w32, w31, w2) -> (w28:errorcluster)
  n114 = Release Notifier(notifier=w25, error in (no error)=w28) -> (error out=w27:errorcluster)  [unwired: 1 in, 2 out]
  n115 = call <vilib>:"General Error Handler.vi"("error in (no error)"=w27) -> ("error out"=w38:errorcluster)  [unwired: 10 in, 4 out]
  n116 = call <vilib>:"Clear Errors.vi"("error in (no error)"=w38) -> ()  [unwired: 5 in, 2 out]
